vi "Create Message Group.vi"(8 "error in (no error)":errorcluster, 10 "message group name":string, 11 "instrument addon refnum in":T1=18446744073709551615 format="%.0x") -> (0 "error out":errorcluster, 2 "message group refnum out":T1=18446744073709551615 format="%.0x", 3 "instrument addon refnum out":T1=18446744073709551615 format="%.0x")   [LabVIEW 2020, in "Instrument Addon Scripting API.lvlib"]
doc: "Creates a new message group section under the Instrument Addon custom device."
uses:
  Instrument Addon Scripting API.lvlib
  <vilib>/NI VeriStand/Custom Device API/Custom Device Item Ref.ctl
  Addon/Addon Shared/SubVIs/Constants.vi
  <vilib>/NI VeriStand/Custom Device API/Custom Device API.lvlib
  Addon/Addon Shared/Instrument Addon Shared.lvlib
  <vilib>/NI VeriStand/Custom Device Tools/Custom Device Utility Library/Custom Device Utility Library.lvlib
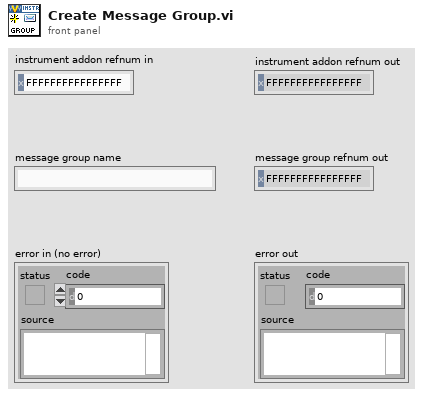
[diagram p1: front panel]
types:
  T1 = typedef "Custom Device API.lvlib/Custom Device Item Ref.ctl" = u64
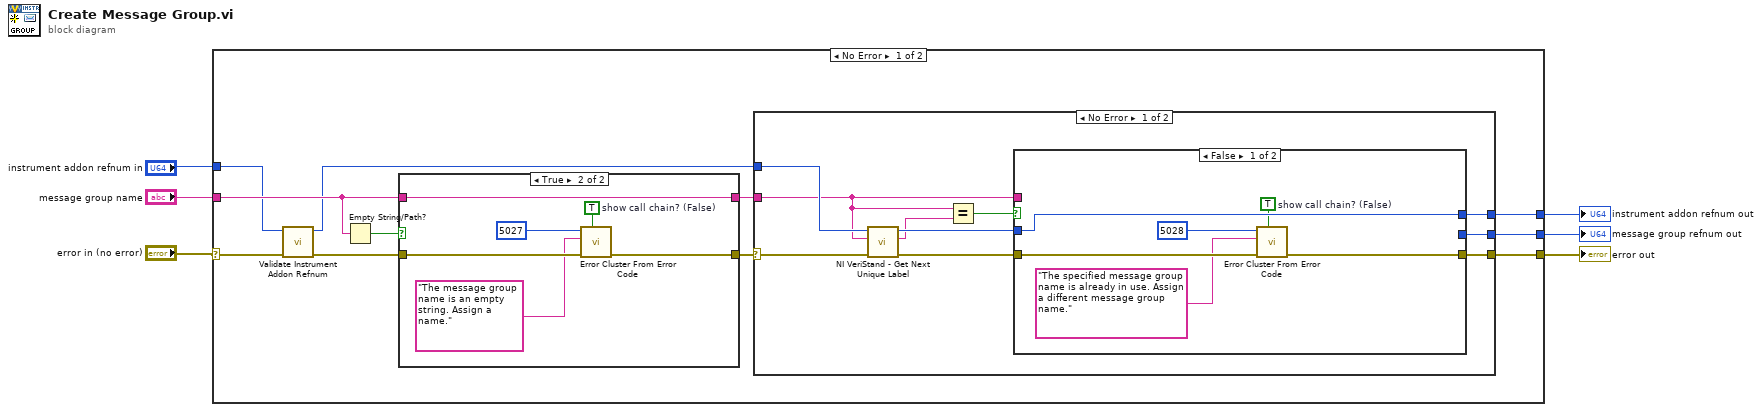
[diagram p0: block diagram]
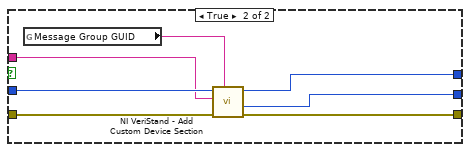
[diagram p2: hidden frame]
diagram:
  n1 = case shown="No Error" "error in (no error)" {
    selector: "error in (no error)" -> [w8 w52]
    tunnel: "message group name" -> [w14 _]
    tunnel: "instrument addon refnum in" -> [w10 w51]
    tunnel: [w17 w52] -> w5
    tunnel: [w11 _] -> w2
    tunnel: [w16 w51] -> w3
    frame No Error {
      n2 = call "Validate Instrument Addon Refnum.vi"("Error In"=w8, "Refnum In"=w10) -> ("Error Out"=w7:errorcluster, "Refnum Out"=w9:T1)  [unwired: 7 in, 1 out]
      n3 = Empty String/Path?(string/path=w14) -> (empty?=w15:bool)
      n4 = case shown="True" w15 {
        tunnel: w7 -> [w44 w49]
        tunnel: [w44 w48] -> w12
        tunnel: w14 -> [w43 w50]
        tunnel: [w43 w50] -> w13
        frame False {
        }
        frame True {
          w46 = TRUE  # show call chain? (False)
          n5 = call <vilib>:"Error Cluster From Error Code.vi"("show call chain? (False)"=w46, "error in (no error)"=w49, "error message (\"\")"="The message group name is an empty string. Assign a name." ("error message (\"\")"), "error code (0)"=5027) -> ("error out"=w48:errorcluster)  [unwired: 5 in]
        }
      }
      n6 = case shown="No Error" w12 {
        selector: w12 -> [w21 w42]
        tunnel: [w27 w42] -> w17
        tunnel: [w26 _] -> w11
        tunnel: [w25 w41] -> w16
        tunnel: w9 -> [w22 w41]
        tunnel: w13 -> [w18 _]
        frame No Error {
          n7 = call <vilib>:"NI VeriStand - Get Next Unique Label.vi"("error in (no error)"=w21, "Label"=w18, "Parent Ref in"=w22) -> ("error out"=w23:errorcluster, "Label out"=w20:string, "Parent Ref dup"=w24:T1)  [unwired: 5 in, 1 out]
          n8 = Equal?(x=w18, y=w20) -> (x = y?=w19:bool)
          n9 = case shown="False" w19 {
            tunnel: [w31 w40] -> w27
            tunnel: [_ w39] -> w26
            tunnel: [w33 w38] -> w25
            tunnel: w24 -> [w33 w37]
            tunnel: w23 -> [w32 w36]
            tunnel: w18 -> [_ w34]
            frame False {
              w29 = TRUE  # show call chain? (False)
              n10 = call <vilib>:"Error Cluster From Error Code.vi"("show call chain? (False)"=w29, "error in (no error)"=w32, "error message (\"\")"="The specified message group name is already in use. Assign a different message group name." ("error message (\"\")"), "error code (0)"=5028) -> ("error out"=w31:errorcluster)  [unwired: 5 in]
            }
            frame True {
              n11 = global read "Constants.vi" "Message Group GUID"() -> (w35:string)
              n12 = call <vilib>:"NI VeriStand - Add Custom Device Section.vi"("GUID (Default Section)"=w35, "error in (no error)"=w36, "Section Name"=w34, "Parent Ref in"=w37) -> ("error out"=w40:errorcluster, "Section Ptr"=w39:T1, "Parent Ref out"=w38:T1)  [unwired: 4 in, 1 out]
            }
          }
        }
        frame Error {
        }
      }
    }
    frame Error {
    }
  }
  "error out" <- w5
  "instrument addon refnum out" <- w3
  "message group refnum out" <- w2
